vi "Scale Value (Power).vi"(11 "Value":dbl) -> (3 "Scaled Value":dbl)   [LabVIEW 2018, in "Audio Processing.lvlib"]
doc: "Scales the input value from range 0-1 to 0-20000, applying an exponential curve."
uses:
  Audio Processing.lvlib
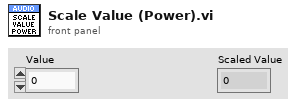
[diagram p1: front panel]
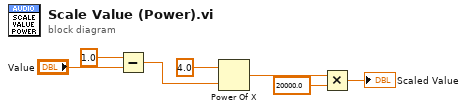
[diagram p0: block diagram]
diagram:
  n1 = Subtract(x=1.0, y="Value") -> (x-y=w3:dbl)
  n2 = Power Of X(1:w3, 2:4.0 ("y")) -> (0:w1:dbl)
  n3 = Multiply(x=w1, y=20000.0) -> (x*y=→"Scaled Value":dbl)
